vi "Main.vi"() -> ()   [LabVIEW 2010]
doc: "Use this template to build a producer/consumer design pattern with events to produce queue items. Use this design pattern instead of the User Interface Event Handler pattern for user interfaces when you want to execute code asynchronously in response to an event without slowing the user interface responsiveness."
uses:
  typedefs/stim_protocol_cluster.ctl
  typedefs/main_state_enum.ctl
  <vilib>/Utility/error.llb/DialogType.ctl
  <vilib>/DAQmx/write.llb/DAQmx Write (Analog 1D DBL 1Chan NSamp).vi
  <vilib>/daqmx/miscellaneous.llb/DAQmx Fill In Error Info.vi
panel:
  in  "Stim protocol":T1={"Frequency"=0.01, "Pulse duration"=0.001, "Stop after"=0.0} {"Stop after" min=0.0 max=500.0; "Pulse duration" min=0.001 max=0.1; "Frequency" min=0.01 max=200.0 step=1.0}
  in  "Run":bool
  in  "Quit":bool
  # "Alberto's ChR2-Stimulator"
  # "0 for manual stop"
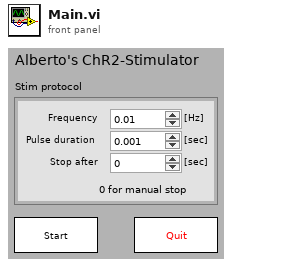
[diagram p1: front panel]
types:
  T1 = typedef "stim_protocol_cluster.ctl" = cluster{"Frequency":dbl, "Pulse duration":dbl, "Stop after":dbl}
  T2 = typedef "DialogType.ctl" = u16
  T3 = typedef "main_state_enum.ctl" = enum16{"Init", "Quit", "Error", "Start", "Stop", "ParamsChanged"}
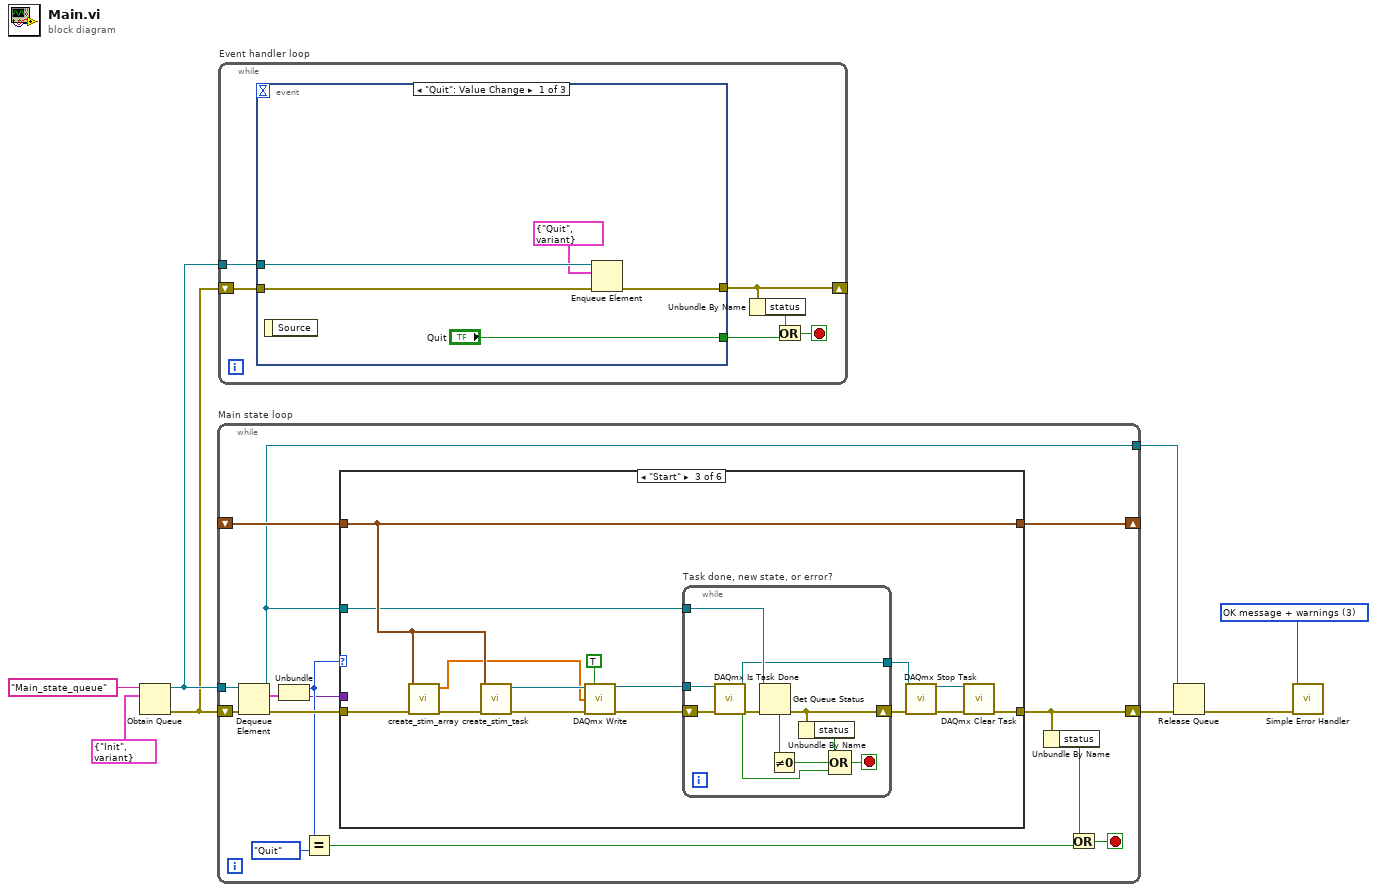
[diagram p0: block diagram]
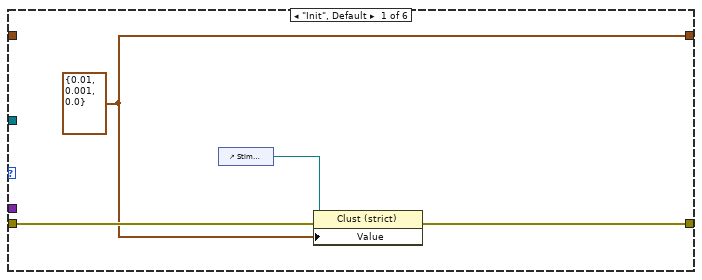
[diagram p2: hidden frame]
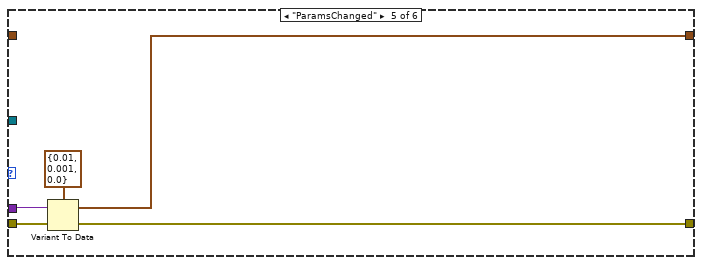
[diagram p5: hidden frame]
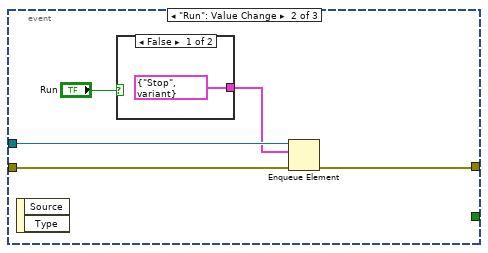
[diagram p7: hidden frame]
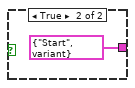
[diagram p8: hidden frame]
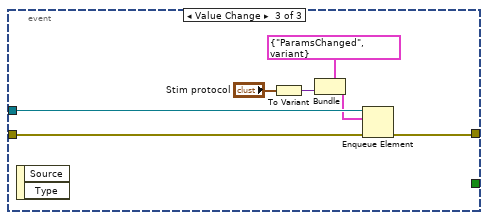
[diagram p9: hidden frame]
diagram:
  w1 = T2 3 items=["no dialog", "OK message", "continue or stop message", "OK message + warnings", "continue/stop + warnings"] ("type of dialog (OK msg:1)")
  n1 = Obtain Queue(name (unnamed)="Main_state_queue", element data type=cluster{"Main state enum":T3, "variant":variant} {"Main state enum"=enum."Init", "variant"=variant}) -> (queue out=w8:refnum<queue>, error out=w7:errorcluster)  [unwired: 3 in, 1 out]
  n2 = while "Main state loop" {
    tunnel: w8 -> [w10]
    shift-right: [w17] -> w4
    shift-left: w7 -> [w22]
    shift-right: [w12] -> _
    shift-left: _ -> [w11]
    tunnel: [w9] -> w3
    stop <- w14 stop-if-true
    n3 = Dequeue Element(queue=w10, error in (no error)=w22) -> (queue out=w9:refnum<queue>, element=w20:cluster{"Main state enum":T3, "variant":variant}, error out=w21:errorcluster)  [unwired: 1 in, 1 out]
    n4 = Unbundle(w20) -> ("Main state enum"=w19:T3, "variant"=w13:variant)
    n5 = Equal?(x=w19, y=main_state_enum."Quit") -> (x = y?=w15:bool)
    n6 = case shown="\"Start\"" w19 {
      tunnel: w21 -> [w26 w28 w42 w56 w61 w63]
      tunnel: [w25 w28 w29 w56 w60 w63] -> w17
      tunnel: w13 -> [_ _ _ _ w59 _]
      tunnel: [w23 w27 w43 w55 w57 w62] -> w12
      tunnel: w11 -> [_ w27 w43 w55 _ w62]
      tunnel: w9 -> [_ _ w34 _ _ _]
      frame "Init", Default {
        w23 = T1 {"Frequency"=0.01, "Pulse duration"=0.001, "Stop after"=0.0} ("Stim protocol")
        n7 = control-ref of="Stim protocol"() -> (w24:refnum<vi>)
        n8 = property class="Clust (strict)"(reference=w24, error in=w26, "Value"=w23) -> (error out=w25:errorcluster)  [unwired: 1 out]
      }
      frame "Error" {
      }
      frame "Start" {
        n9 = call "create_stim_array.vi"("error in"=w42, "Stim protocol"=w43) -> ("error out"=w38:errorcluster, "Stim array"=w39:dbl[])  [unwired: 8 in]
        n10 = call "create_stim_task.vi"("error in"=w38, "Stim protocol"=w43) -> ("error out"=w41:errorcluster, "task out"=w40:refnum<k21>)  [unwired: 8 in]
        n11 = call-poly <vilib>:"DAQmx Write.vi"("task/channels in"=w40, "auto start"=TRUE, "data"=w39, "error in"=w41) -> ("task out"=w35:refnum<k21>, "error out"=w36:errorcluster)  [unwired: 9 in, 1 out]
        n12 = while "Task done, new state, or error?" {
          shift-right: [w50] -> w32
          shift-left: w36 -> [w54]
          tunnel: w35 -> [w53]
          tunnel: w34 -> [w51]
          tunnel: [w44] -> w33
          stop <- w49 stop-if-true
          n13 = call <vilib>:"DAQmx Is Task Done.vi"("task/channels in"=w53, "error in"=w54) -> ("task out"=w44:refnum<k21>, "task done?"=w45:bool, "error out"=w52:errorcluster)  [unwired: 11 in]
          n14 = Get Queue Status(queue=w51, error in (no error)=w52) -> (error out=w50:errorcluster, # elements in queue=w46:i32)  [unwired: 1 in, 6 out]
          n15 = Not Equal To 0?(x=w46) -> (x != 0?=w47:bool)
          n16 = Unbundle By Name(w50) -> ("status"=w48:bool)
          n17 = Compound Arithmetic op=OR(w48, w47, w45) -> (w49:bool)
        }
        n18 = call <vilib>:"DAQmx Stop Task.vi"("task/channels in"=w33, "error in"=w32) -> ("task out"=w31:refnum<k21>, "error out"=w30:errorcluster)  [unwired: 12 in]
        n19 = call <vilib>:"DAQmx Clear Task.vi"("task in"=w31, "error in"=w30) -> ("error out"=w29:errorcluster)  [unwired: 13 in]
      }
      frame "Stop" {
      }
      frame "ParamsChanged" {
        n20 = Variant To Data(error in=w61, Variant=w59, type=T1 {"Frequency"=0.01, "Pulse duration"=0.001, "Stop after"=0.0} ("Stim protocol")) -> (error out=w60:errorcluster, data=w57:T1)
      }
      frame "Quit" {
      }
    }
    n21 = Unbundle By Name(w17) -> ("status"=w16:bool)
    n22 = Or(x=w16, y=w15) -> (x .or. y?=w14:bool)
  }
  n23 = while "Event handler loop" {
    shift-right: [w65] -> _
    shift-left: w7 -> [w68]
    tunnel: w8 -> [w69]
    stop <- w66 stop-if-true
    n24 = event shown="[0] \"Quit\": Value Change" {
      selector: _ -> [_ _ _]
      dyn-events: _ -> [_ _ _]
      timeout: _ -> [_ _ _]
      tunnel: w69 -> [w71 w77 w86]
      tunnel: w68 -> [w73 w79 w88]
      tunnel: [w72 w78 w87] -> w65
      tunnel: ["Quit" _ _] -> w67
      event "Quit": Value Change {
        n25 = event-data() -> ()  [unwired: 1 in, 1 out]
        n26 = Enqueue Element(queue=w71, element=cluster{"Main state enum":T3, "variant":variant} {"Main state enum"=enum."Quit", "variant"=variant}, error in (no error)=w73) -> (error out=w72:errorcluster)  [unwired: 1 in, 2 out]
      }
      event "Run": Value Change {
        n27 = event-data() -> ()  [unwired: 1 in, 2 out]
        n28 = case shown="False" "Run" {
          tunnel: [cluster{"Main state enum":T3, "variant":variant} {"Main state enum"=enum."Stop", "variant"=variant} ("element") cluster{"Main state enum":T3, "variant":variant} {"Main state enum"=enum."Start", "variant"=variant} ("element")] -> w75
          frame False {
          }
          frame True {
          }
        }
        n29 = Enqueue Element(queue=w77, element=w75, error in (no error)=w79) -> (error out=w78:errorcluster)  [unwired: 1 in, 2 out]
      }
      event Value Change {
        n30 = event-data() -> ()  [unwired: 1 in, 2 out]
        n31 = To Variant(anything="Stim protocol") -> (Variant=w83:variant)
        n32 = Bundle(cluster=cluster{"Main state enum":T3, "variant":variant} {"Main state enum"=enum."ParamsChanged", "variant"=variant} ("element"), "variant"=w83) -> (w85:cluster{"Main state enum":T3, "variant":variant})  [unwired: 1 in]
        n33 = Enqueue Element(queue=w86, element=w85, error in (no error)=w88) -> (error out=w87:errorcluster)  [unwired: 1 in, 2 out]
      }
    }
    n34 = Unbundle By Name(w65) -> ("status"=w64:bool)
    n35 = Or(x=w64, y=w67) -> (x .or. y?=w66:bool)
  }
  n36 = Release Queue(queue=w3, error in (no error)=w4) -> (error out=w2:errorcluster)  [unwired: 1 in, 2 out]
  n37 = call <vilib>:"Simple Error Handler.vi"("type of dialog (OK msg:1)"=w1, "error in (no error)"=w2) -> ()  [unwired: 3 in, 5 out]
